vi "test-Rect-Region-Constraint-Test2.vi"(8 "error in (no error)":errorcluster) -> (0 "error out":errorcluster, 3 "All tests passed":bool)   [LabVIEW 2019]
uses:
  <vilib>/Rock Robotics/WPI/ThirdParty/JAS_Junk/TrajLib/TypeDef/TRAJ_CONSTRAINT_RECT_REGION.ctl
  <vilib>/Rock Robotics/WPI/ThirdParty/JAS_Junk/TrajLib/TRANSLATION2D.ctl
  <vilib>/Rock Robotics/WPI/ThirdParty/JAS_Junk/TrajLib/Enum/TRAJ_CONSTRAINT_TYPES_ENUM.ctl
  <vilib>/Rock Robotics/WPI/ThirdParty/JAS_Junk/TrajLib/Rotation2d_CreateAngle.vi
  <vilib>/Rock Robotics/WPI/ThirdParty/JAS_Junk/TrajLib/VI/TrajConstraint_GetType.vi
  <vilib>/Utility/Data Type/Get Type Information.vi
  <vilib>/Rock Robotics/WPI/ThirdParty/JAS_Junk/TrajLib/Trajectory_Library.lvlib
panel:
  out "RECT_REGION_CONSTRAINT":T1={"BottomLeftPoint"={"X"=0.0, "Y"=0.0}, "TopRightPoint"={"X"=0.0, "Y"=0.0}, "Constraint"=variant, "Constraint Type"=enum."DIFF DRIVE KINEMATICS"} {"TopRightPoint"."Y" format="%14.3f"; "TopRightPoint"."X" format="%14.3f"; "BottomLeftPoint"."Y" format="%14.3f"; "BottomLeftPoint"."X" format="%14.3f"}
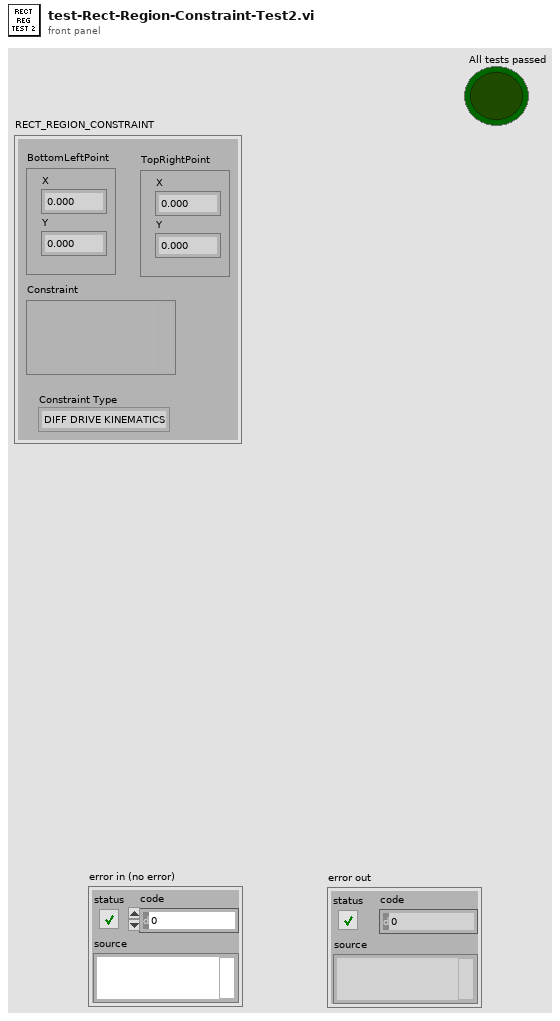
[diagram p1: front panel]
types:
  T1 = typedef "Trajectory_Library.lvlib/TRAJ_CONSTRAINT_RECT_REGION.ctl" = cluster{"BottomLeftPoint":T2, "TopRightPoint":T2, "Constraint":variant, "Constraint Type":T3}
  T2 = typedef "Trajectory_Library.lvlib/TRANSLATION2D.ctl" = cluster{"X":dbl, "Y":dbl}
  T3 = typedef "Trajectory_Library.lvlib/TRAJ_CONSTRAINT_TYPES_ENUM.ctl" = enum16{"UNDEFINED", "DIFF DRIVE KINEMATICS", "DIFF DRIVE VOLTAGE", "CENTRIPITAL ACCEL", "MECA DRIVE KINEMATICS", "SWERVE DRIVE KINEMATICS", "MAXIMUM VELOCITY"}
  T4 = typedef "Trajectory_Library.lvlib/TRAJ_CONSTRAINT_MAX_VELOCITY.ctl" = cluster{"Max Velocity":dbl, "IM UNIQUE":bool}
  T5 = typedef "Trajectory_Library.lvlib/POSE2D.ctl" = cluster{"TRANSLATION":T2, "ROTATION":T6}
  T6 = typedef "Trajectory_Library.lvlib/ROTATION2D.ctl" = cluster{"VALUE":dbl, "COS":dbl, "SIN":dbl}
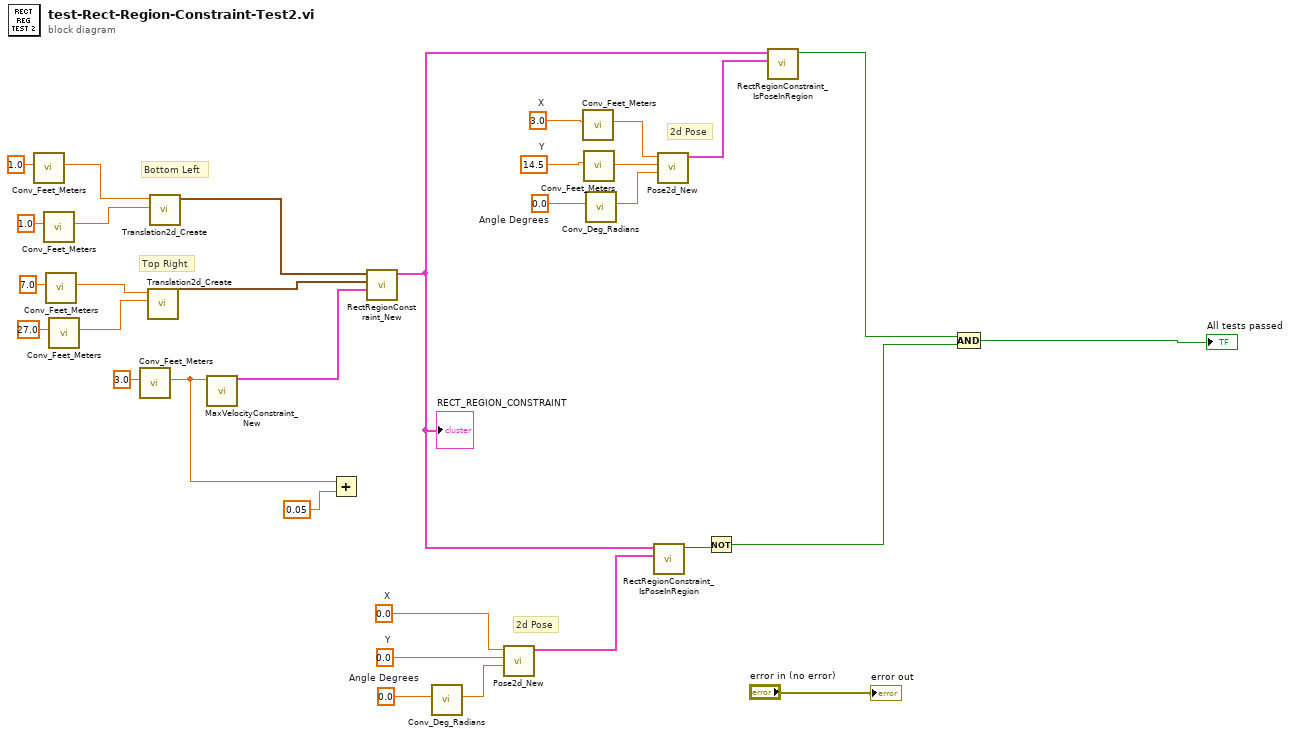
[diagram p0: block diagram]
diagram:
  w6 = 3.0  # X
  w5 = 14.5  # Y
  w9 = 0.0  # Angle Degrees
  w16 = 0.0  # X
  w15 = 0.0  # Y
  w13 = 0.0  # Angle Degrees
  # "2d Pose"
  # "2d Pose"
  # "Top Right"
  # "Bottom Left"
  n1 = call <vilib>:"Conv_Feet_Meters.vi"("Feet"=1.0) -> ("Meters"=w23:dbl)  [unwired: 10 in]
  n2 = call <vilib>:"Conv_Feet_Meters.vi"("Feet"=1.0) -> ("Meters"=w22:dbl)  [unwired: 10 in]
  n3 = call <vilib>:"Conv_Feet_Meters.vi"("Feet"=7.0) -> ("Meters"=w21:dbl)  [unwired: 10 in]
  n4 = call <vilib>:"Conv_Feet_Meters.vi"("Feet"=27.0) -> ("Meters"=w20:dbl)  [unwired: 10 in]
  n5 = call <vilib>:"Conv_Feet_Meters.vi"("Feet"=3.0) -> ("Meters"=w19:dbl)  [unwired: 10 in]
  n6 = call <vilib>:"Translation2d_Create.vi"("Y"=w20, "X"=w21) -> ("TRANSLATION"=w29:T2)  [unwired: 9 in]
  n7 = call <vilib>:"Translation2d_Create.vi"("Y"=w22, "X"=w23) -> ("TRANSLATION"=w30:T2)  [unwired: 9 in]
  n8 = call <vilib>:"MaxVelocityConstraint_New.vi"("Maximum Velocity"=w19) -> ("MAX_VELOCITY_CONSTRAINT"=w28:T4)  [unwired: 10 in]
  n9 = Add(x=w19, y=0.05) -> ()  [unwired: 1 out]
  n10 = call <vilib>:"RectRegionConstraint_New.vi"("Constraint Data Cluster"=w28, "TopRightPoint"=w29, "BottomLeftPoint"=w30) -> ("RECT_REGION_CONSTRAINT"=w8:T1)  [unwired: 8 in]
  "RECT_REGION_CONSTRAINT" <- w8
  n11 = call <vilib>:"Conv_Deg_Radians.vi"("Degress"=w13) -> ("Radians"=w14:dbl)  [unwired: 10 in]
  n12 = call <vilib>:"Pose2d_New.vi"("Heading"=w14, "Y"=w15, "X"=w16) -> ("out POSe"=w12:T5)  [unwired: 8 in]
  n13 = call <vilib>:"Conv_Feet_Meters.vi"("Feet"=w6) -> ("Meters"=w4:dbl)  [unwired: 10 in]
  n14 = call <vilib>:"Conv_Feet_Meters.vi"("Feet"=w5) -> ("Meters"=w3:dbl)  [unwired: 10 in]
  n15 = call <vilib>:"Conv_Deg_Radians.vi"("Degress"=w9) -> ("Radians"=w10:dbl)  [unwired: 10 in]
  n16 = call <vilib>:"RectRegionConstraint_IsPoseInRegion.vi"("statePose"=w12, "RECT_REGION_CONSTRAINT"=w8) -> ("PoseInRegion"=w11:bool)  [unwired: 9 in]
  n17 = call <vilib>:"Pose2d_New.vi"("Heading"=w10, "Y"=w3, "X"=w4) -> ("out POSe"=w7:T5)  [unwired: 8 in]
  n18 = Not(x=w11) -> (.not. x?=w1:bool)
  n19 = call <vilib>:"RectRegionConstraint_IsPoseInRegion.vi"("statePose"=w7, "RECT_REGION_CONSTRAINT"=w8) -> ("PoseInRegion"=w2:bool)  [unwired: 9 in]
  n20 = Compound Arithmetic op=AND(w2, w1) -> (→"All tests passed":bool)
  "error out" <- "error in (no error)"
